vi "oa_Adjust Resample State Info.vi"(7 "Reset? (True)":bool=TRUE, 10 "time position":dbl[](array[numeric]), 11 "state in":T1 {"time interval" format="%.2f"; "position" format="%.2f"; "init condition" format="%.2f"}) -> (2 "reset pending":bool, 3 "state out":T1 {"time interval" format="%.2f"; "position" format="%.2f"; "init condition" format="%.2f"})   [LabVIEW 2017, in "SoundVib_Resampling.lvlib"]
uses:
  <vilib>/addons/Sound and Vibration/Order Analysis/Resample Order Tracking/SoundVib_Resampling.lvlib
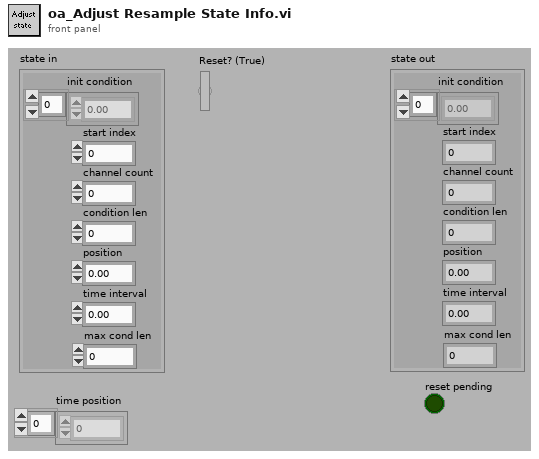
[diagram p1: front panel]
types:
  T1 = cluster{"init condition":dbl[], "start index":i32, "channel count":i32, "condition len":i32, "position":dbl, "time interval":dbl, "max cond len":i32}
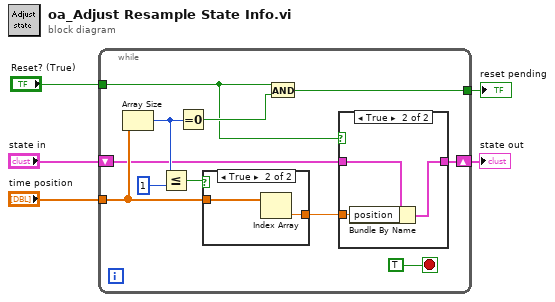
[diagram p0: block diagram]
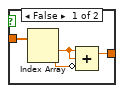
[diagram p3: hidden frame]
diagram:
  n1 = while {
    tunnel: "time position" -> [w14]
    tunnel: "Reset? (True)" -> [w6]
    tunnel: [w15] -> w1
    shift-right: [w9] -> w2
    shift-left: "state in" -> [w7]
    stop <- TRUE stop-if-true
    n2 = Array Size(array=w14) -> (size(s)=w12:i32)
    n3 = Less Or Equal?(x=w12, y=1) -> (x <= y?=w13:bool)
    n4 = Equal To 0?(x=w12) -> (x = 0?=w10:bool)
    n5 = case shown="True" w13 {
      tunnel: [w23 w26] -> w8
      tunnel: w14 -> [w24 w25]
      frame False {
        n6 = Index Array(array=w24) -> (element #1=w22:dbl, element #2=w21:dbl)  [unwired: 2 in]
        n7 = Compound Arithmetic op=ADD(w22, w22, invert w21) -> (w23:dbl)
      }
      frame True {
        n8 = Index Array(array=w25) -> (element=w26:dbl)  [unwired: 1 in]
      }
    }
    n9 = And(x=w6, y=w10) -> (x .and. y?=w15:bool)
    n10 = case shown="True" w6 {
      tunnel: w7 -> [w17 w20]
      tunnel: w8 -> [_ w19]
      tunnel: [w17 w18] -> w9
      frame False {
      }
      frame True {
        n11 = Bundle By Name(cluster=w20, "position"=w19) -> (w18:T1)
      }
    }
  }
  "state out" <- w2
  "reset pending" <- w1
